vi "3DSim2.0.vi"() -> ()   [LabVIEW 2024]
uses:
  <vilib>/Analysis/Matrix/Datatypes/RealMatrix.ctl
  <vilib>/Utility/miscctls.llb/LV3DPointTypeDef.ctl
  <vilib>/Analysis/baseanly.llb/Real A x B.vi
  <vilib>/Analysis/NI_AALBase.lvlib
  <vilib>/Analysis/Matrix/NI_Matrix.lvlib
panel:
  out "3D Picture 2":refnum<vi>(3d-picture)
  in  "Joints":T1(array[cluster])=[{"Theta"=0.0, "Translation"={"X"=0.0, "Y"=0.0, "Z"=0.0}, "Axis"=enum."z"}] {"Theta" scale=-180.0..180.0}
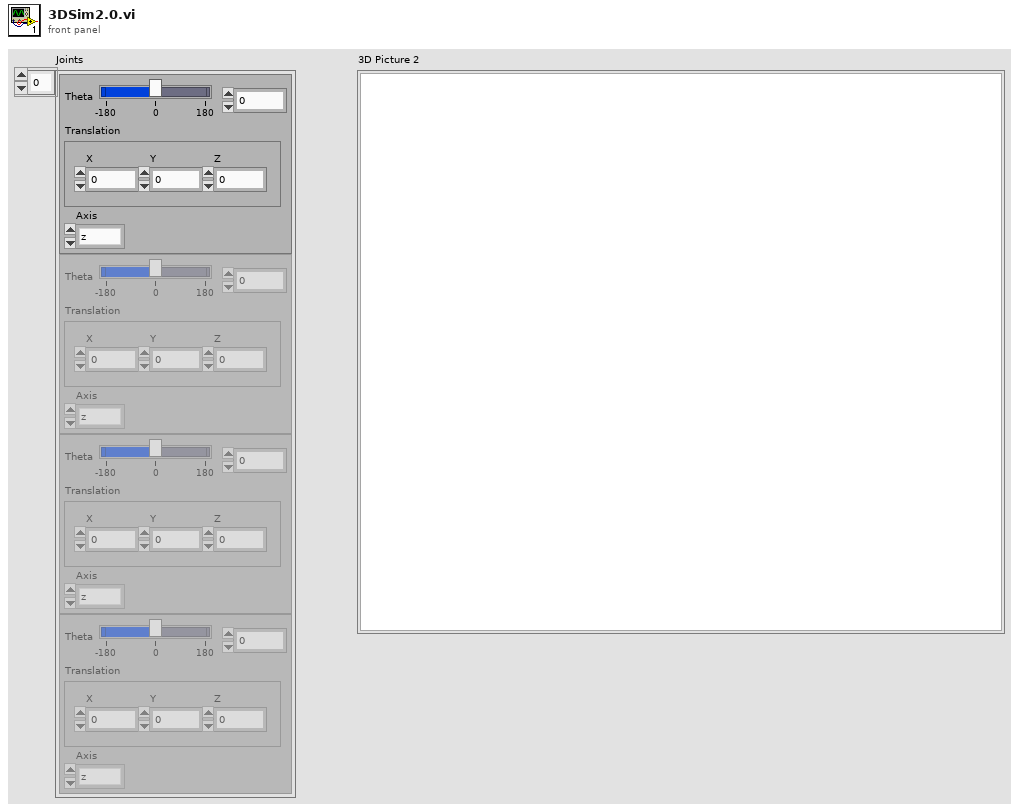
[diagram p1: front panel]
types:
  T1 = cluster{"Theta":dbl, "Translation":cluster{"X":dbl, "Y":dbl, "Z":dbl}, "Axis":enum16{"x", "y", "z"}}[]
  T2 = typedef "LV3DPointTypeDef.ctl" = cluster{"X":sgl, "Y":sgl, "Z":sgl}
  T3 = enum16{"None", "Spherical", "Flying", "Oriented"}
  T4 = typedef "NI_Matrix.lvlib/RealMatrix.ctl" = dbl[][]
  T5 = cluster{"Line width":sgl, "Line Color":u32, "Axes?":bool}
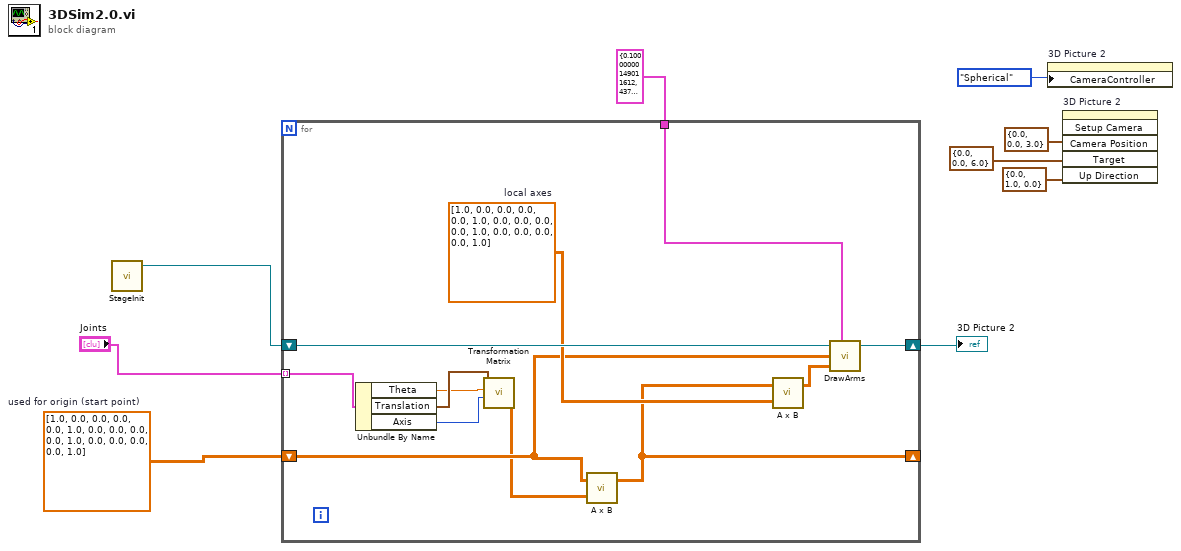
[diagram p0: block diagram]
diagram:
  w7 = T4 [[1.0, 0.0, 0.0, 0.0], [0.0, 1.0, 0.0, 0.0], [0.0, 0.0, 1.0, 0.0], [0.0, 0.0, 0.0, 1.0]]  # used for origin (start point)
  n1 = call "StageInit.vi"() -> ("Stage out"=w6:refnum<vi>)  [unwired: 4 in, 1 out]
  n2 = for {
    tunnel: "Joints" -> [w14] mode=indexing
    tunnel: T5 {"Line width"=0.1, "Line Color"=4376575, "Axes?"=TRUE} ("Params") -> [w21]
    shift-right: [w11] -> _
    shift-left: w7 -> [w13]
    shift-right: [w19] -> w5
    shift-left: w6 -> [w20]
    w18 = T4 [[1.0, 0.0, 0.0, 0.0], [0.0, 1.0, 0.0, 0.0], [0.0, 0.0, 1.0, 0.0], [0.0, 0.0, 0.0, 1.0]]  # local axes
    n3 = Unbundle By Name(w14) -> ("Theta"=w15:dbl, "Translation"=w16:cluster{"X":dbl, "Y":dbl, "Z":dbl}, "Axis"=w10:enum16{"x", "y", "z"})
    n4 = call "Transformation Matrix.vi"("Axis"=w10, "Angle (degrees)"=w15, "Translation"=w16) -> ("Transformation Matrix"=w12:T4)  [unwired: 8 in]
    n5 = call-poly <vilib>:"A x B.vi"("B"=w12, "A"=w13) -> ("A x B"=w11:T4)  [unwired: 1 out]
    n6 = call-poly <vilib>:"A x B.vi"("B"=w18, "A"=w11) -> ("A x B"=w17:T4)  [unwired: 1 out]
    n7 = call "DrawArms.vi"("Stage in"=w20, "Params"=w21, "Start"=w13, "End"=w17) -> ("Stage out"=w19:refnum<vi>)  [unwired: 2 in, 1 out]
  }
  "3D Picture 2" <- w5
  n8 = property on="3D Picture 2" class="SceneGraphDisp (strict)"("CameraController"=T3."Spherical" ("Camera Controller:Type")) -> ()  [unwired: 2 in, 2 out]
  n9 = invoke on="3D Picture 2" class="SceneGraphDisp (strict)" method="Setup Camera"("Camera Position"=T2 {"X"=0.0, "Y"=0.0, "Z"=6.0}, "Target"=T2 {"X"=0.0, "Y"=0.0, "Z"=3.0}, "Up Direction"=T2 {"X"=0.0, "Y"=1.0, "Z"=0.0}) -> ()  [unwired: 3 in, 6 out]
